vi "Current State.vi"(8 "error in (no error)":errorcluster, 10 "StateState":T1, 11 "Receiver in":refnum<class "Receiver.lvclass">) -> (0 "error out":errorcluster, 3 "Receiver out":refnum<class "Receiver.lvclass">)   [LabVIEW 2013]
uses:
  Receiver.lvclass
  ReceiverState/StateState.ctl
  Connect Command/Connect Command.lvclass
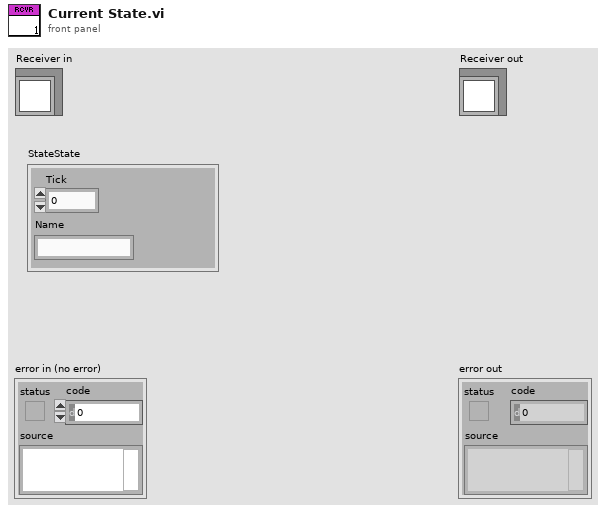
[diagram p1: front panel]
types:
  T1 = typedef "Receiver.lvlib/Receive Commands Using State Actors.lvlib/Connect Command.lvlib/Connect Command.lvclass/StateState.ctl" = cluster{"Tick":u32, "Name":string}
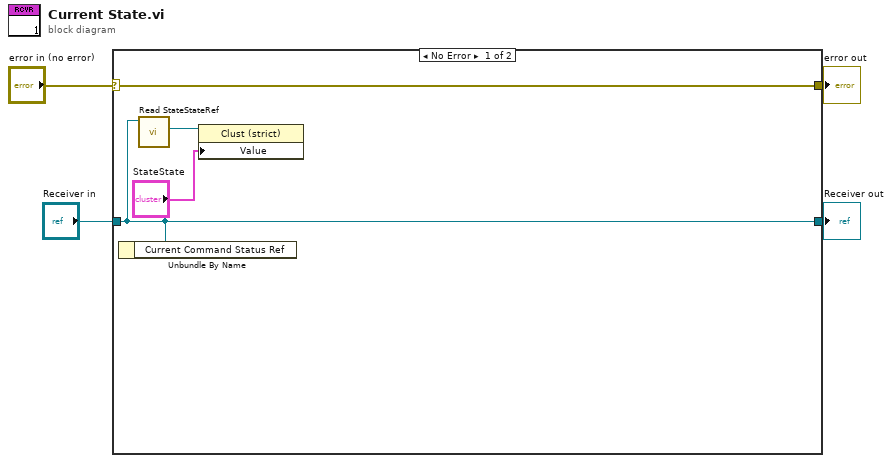
[diagram p0: block diagram]
diagram:
  n1 = case shown="No Error" "error in (no error)" {
    selector: "error in (no error)" -> [w8 w10]
    tunnel: [w8 w10] -> w3
    tunnel: [w5 w9] -> w1
    tunnel: "Receiver in" -> [w5 w9]
    frame No Error {
      n2 = Unbundle By Name(w5) -> ()  [unwired: 1 out]
      n3 = call-dynamic "Read StateStateRef.vi"("Receiver in"=w5) -> ("StateStateRef"=w7:refnum<vi>)  [unwired: 8 in, 2 out]
      n4 = property class="Clust (strict)"(reference=w7, "Value"="StateState") -> ()  [unwired: 1 in, 2 out]
    }
    frame Error {
    }
  }
  "error out" <- w3
  "Receiver out" <- w1
